vi "Set Displayed Sequence.vi"(8 "error in (no error)":errorcluster, 10 "Sequence Name":string, 11 "SequenceViewPanel in":refnum<class "SequenceViewPanel.lvclass">) -> (0 "error out":errorcluster, 3 "SequenceViewPanel out":refnum<class "SequenceViewPanel.lvclass">)   [LabVIEW 2020, in "TSnax UI.lvlib" / "SequenceViewPanel.lvclass"]
uses:
  SequenceViewPanel.lvclass
  SequenceViewPanel.lvclass/SequenceViewPanel.ctl
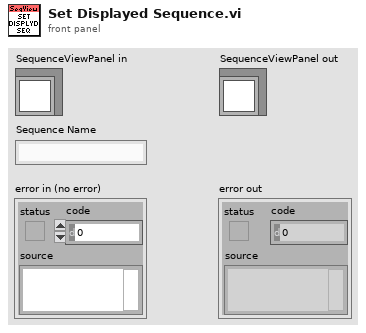
[diagram p1: front panel]
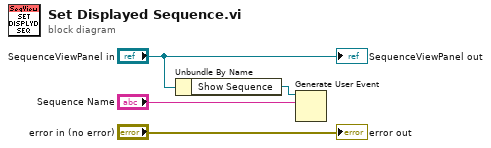
[diagram p0: block diagram]
diagram:
  n1 = Unbundle By Name("SequenceViewPanel in") -> ("Show Sequence"=w2:refnum<user-event>)
  n2 = Generate User Event(user event=w2, event data cluster="Sequence Name") -> ()  [unwired: 2 in, 2 out]
  "error out" <- "error in (no error)"
  "SequenceViewPanel out" <- "SequenceViewPanel in"
